vi "Drive_Open4CANMotor.vi"(8 "RightSlaveID":u8, 9 "RightMasterID":u8, 10 "LeftSlaveID":u8, 11 "LeftMasterID":u8) -> ()   [LabVIEW 2017]
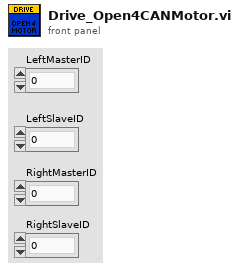
[diagram p1: front panel]
types:
  T1 = typedef "WPI_MotorControlDeviceRef.ctl" = cluster{"DeviceStatus":errorcluster, "Type":T2, "PWM":cluster{"PWM Channel":T3, "DeadBand":T4}, "CAN":cluster{"Device Number":u8, "SetOutput VI Ref":variant, "GetOutput VI Ref":variant, "Enable VI Ref":variant, "Disable VI Ref":variant, "Data":variant}, "Invert":bool, "DIO PWM":cluster{"PWM \"Enable\" Channel":T3, "DIOChannel":T5, "PWM Rate":dbl}}
  T2 = typedef "WPI_MotorControlType.ctl" = enum16{"PWM", "CAN", "DIO PWM"}
  T3 = typedef "FPGA_DIOPWMChannel.ctl" = enum8{"PWM 0", "PWM 1", "PWM 2", "PWM 3", "PWM 4", "PWM 5", "PWM 6", "PWM 7", "PWM 8", "PWM 9", "PWM MXP 0", "PWM MXP 1", "PWM MXP 2", "PWM MXP 3", "PWM MXP 4", "PWM MXP 5", "PWM MXP 6", "PWM MXP 7", "PWM MXP 8", "PWM MXP 9", "Invalid"}
  T4 = typedef "WPI_PWMDeadband.ctl" = cluster{"Name":string, "maxPositivePwm":i32, "minPositivePwm":i32, "centerPwm":i32, "maxNegativePwm":i32, "minNegativePwm":i32, "angularRange":u16}
  T5 = typedef "FPGA_DIOChannel.ctl" = enum8{"DIO 0", "DIO 1", "DIO 2", "DIO 3", "DIO 4", "DIO 5", "DIO 6", "DIO 7", "DIO 8", "DIO 9", "DIO MXP 0", "DIO MXP 1", "DIO MXP 2", "DIO MXP 3", "DIO MXP 4", "DIO MXP 5", "DIO MXP 6", "DIO MXP 7", "DIO MXP 8", "DIO MXP 9", "DIO MXP 10", "DIO MXP 11", "DIO MXP 12", "DIO MXP 13", "DIO MXP 14", "DIO MXP 15", "SPI Port CS1", "SPI Port CS2", "SPI Port CS3", "SPI Port MISO", "SPI Port MOSI", "Invalid"}
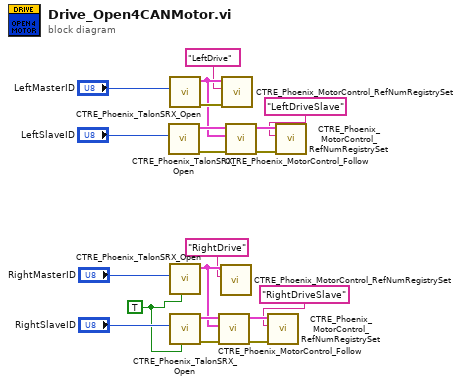
[diagram p0: block diagram]
diagram:
  w1 = TRUE ("Invert")
  n1 = call "CTRE_Phoenix_TalonSRX_Open.vi"("Device Number"="LeftSlaveID") -> ("error out"=w18:errorcluster, "CAN Talon SRX Ref"=w17:T1)  [unwired: 9 in]
  n2 = call "CTRE_Phoenix_TalonSRX_Open.vi"("Device Number"="LeftMasterID") -> ("error out"=w15:errorcluster, "CAN Talon SRX Ref"=w14:T1)  [unwired: 9 in]
  n3 = call "CTRE_Phoenix_TalonSRX_Open.vi"("Invert"=w1, "Device Number"="RightMasterID") -> ("CAN Talon SRX Ref"=w3:T1)  [unwired: 8 in, 1 out]
  n4 = call "CTRE_Phoenix_TalonSRX_Open.vi"("Invert"=w1, "Device Number"="RightSlaveID") -> ("error out"=w8:errorcluster, "CAN Talon SRX Ref"=w7:T1)  [unwired: 8 in]
  n5 = call "CTRE_Phoenix_MotorControl_Follow.vi"("error in (no error)"=w8, "Master Controller to Follow"=w3, "PhoenixMotorControlDevRef"=w7) -> ("error out"=w10:errorcluster, "PhoenixMotorControlDevRef"=w9:T1)  [unwired: 7 in]
  n6 = call "CTRE_Phoenix_MotorControl_RefNumRegistrySet.vi"("refnum name"="RightDrive", "PhoenixMotorControlDevRef"=w3) -> ()  [unwired: 8 in, 2 out]
  n7 = call "CTRE_Phoenix_MotorControl_RefNumRegistrySet.vi"("error in (no error)"=w15, "refnum name"="LeftDrive", "PhoenixMotorControlDevRef"=w14) -> ()  [unwired: 7 in, 2 out]
  n8 = call "CTRE_Phoenix_MotorControl_Follow.vi"("error in (no error)"=w18, "Master Controller to Follow"=w14, "PhoenixMotorControlDevRef"=w17) -> ("error out"=w20:errorcluster, "PhoenixMotorControlDevRef"=w19:T1)  [unwired: 7 in]
  n9 = call "CTRE_Phoenix_MotorControl_RefNumRegistrySet.vi"("error in (no error)"=w10, "refnum name"="RightDriveSlave", "PhoenixMotorControlDevRef"=w9) -> ()  [unwired: 7 in, 2 out]
  n10 = call "CTRE_Phoenix_MotorControl_RefNumRegistrySet.vi"("error in (no error)"=w20, "refnum name"="LeftDriveSlave", "PhoenixMotorControlDevRef"=w19) -> ()  [unwired: 7 in, 2 out]
